vi "WaveGeneratorSetParameters.vi"(0 "stimulus specifier":T3, 2 "stimulus parameters":T1) -> (3 "stimulus specifier 2":T3, 4 "stimulus information":T2, 5 "stimulus parameters":T1, 6 "error IO":errorcluster)   [LabVIEW 2014]
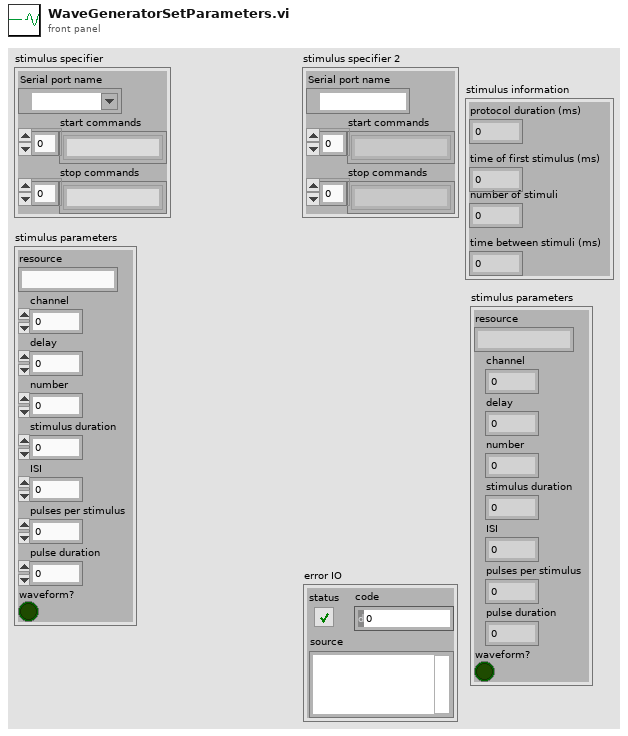
[diagram p1: front panel]
types:
  T1 = cluster{"resource":string, "channel":u16, "delay":dbl, "number":i32, "stimulus duration":dbl, "ISI":dbl, "pulses per stimulus":u16, "pulse duration":dbl, "waveform?":bool}
  T2 = cluster{"protocol duration (ms)":i64, "time of first stimulus (ms)":i64, "number of stimuli":u16, "time between stimuli (ms)":i64}
  T3 = cluster{"Serial port name":refnum<visa-resource-name>, "start commands":string[], "stop commands":string[]}
  T4 = cluster{dbl, "Number\nof stimuli":u16, dbl, dbl, u16}
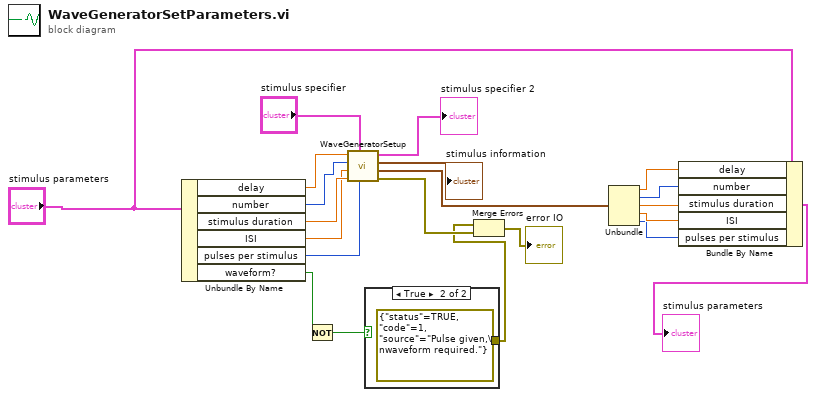
[diagram p0: block diagram]
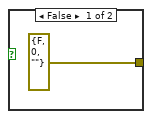
[diagram p2: hidden frame]
diagram:
  n1 = Unbundle By Name("stimulus parameters") -> ("delay"=w16:dbl, "number"=w17:i32, "stimulus duration"=w19:dbl, "ISI"=w18:dbl, "pulses per stimulus"=w20:u16, "waveform?"=w9:bool)
  n2 = Not(x=w9) -> (.not. x?=w10:bool)
  n3 = call "WaveGeneratorSetup.vi"("Frequency"=w20, "stimulus specifier"="stimulus specifier", "Stimulus\nduration (s)"=w19, "Time between stimuli,\nstart-to-start (s)"=w18, "Number\nof stimuli"=w17, "Initial delay (s)"=w16) -> ("error IO"=w13:errorcluster, "stimulus parameters"=w8:T4, "stimulus information"=→"stimulus information":T2, "stimulus specifier"=→"stimulus specifier 2":T3)  [unwired: 2 in]
  n4 = case shown="True" w10 {
    tunnel: [errorcluster {"status"=FALSE, "code"=0, "source"=""} ("error constant") errorcluster {"status"=TRUE, "code"=1, "source"="Pulse given,\nwaveform required."} ("error constant")] -> w12
    frame False {
    }
    frame True {
    }
  }
  n5 = Merge Errors(w12, w13) -> (→"error IO":errorcluster)
  n6 = Unbundle(w8) -> (w6:dbl, "Number\nof stimuli"=w5:u16, w4:dbl, w3:dbl, w2:u16)
  n7 = Bundle By Name(cluster="stimulus parameters", "delay"=w6, "number"=w5, "stimulus duration"=w4, "ISI"=w3, "pulses per stimulus"=w2) -> (→"stimulus parameters":T1)
